vi "Generate External Actuator Channels.vi"() -> (1 "Output Channels":refnum<k21>[](array[refnum]), 3 "Input Channels":refnum<k21>[](array[refnum]))   [LabVIEW 2009]
uses:
  Data Access Objects/Metadata/Persistant DAO Actions.ctl
  Data Access Objects/External Actuators/External Actuator Id.ctl
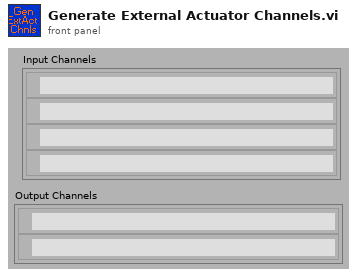
[diagram p1: front panel]
types:
  T1 = typedef "External Actuator Id.ctl" = enum16{"Left", "Right"}
  T2 = typedef "Persistant DAO Actions.ctl" = enum16{"Init", "Get", "Set", "Load", "Save"}
  T3 = typedef "External Actuator Channels.ctl" = cluster{"Load Cell":refnum<k21>, "LVDT":refnum<k21>, "Command":refnum<k21>, "Command\nReturn":refnum<k21>}
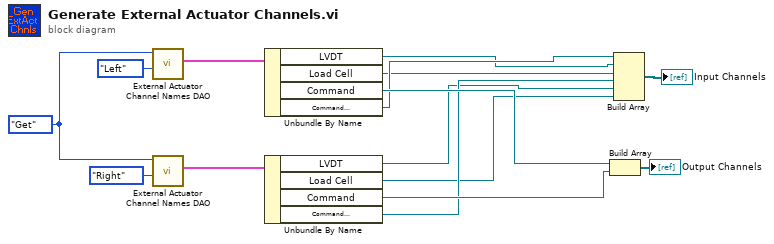
[diagram p0: block diagram]
diagram:
  w11 = Persistant_DAO_Actions."Get" ("Persistent DAO Actions")
  n1 = call "External Actuator Channel Names DAO.vi"("External Actuator Id"=External_Actuator_Id."Left", "Persistent DAO Actions"=w11) -> ("DAQ Channel Out"=w14:T3)  [unwired: 7 in, 2 out]
  n2 = call "External Actuator Channel Names DAO.vi"("External Actuator Id"=External_Actuator_Id."Right", "Persistent DAO Actions"=w11) -> ("DAQ Channel Out"=w12:T3)  [unwired: 7 in, 2 out]
  n3 = Unbundle By Name(w14) -> ("LVDT"=w5:refnum<k21>, "Load Cell"=w4:refnum<k21>, "Command"=w10:refnum<k21>, "Command\nReturn"=w6:refnum<k21>)
  n4 = Unbundle By Name(w12) -> ("LVDT"=w2:refnum<k21>, "Load Cell"=w1:refnum<k21>, "Command"=w9:refnum<k21>, "Command\nReturn"=w3:refnum<k21>)
  n5 = Build Array(w10, w9) -> (→"Output Channels":refnum<k21>[])
  n6 = Build Array(w6, w5, w4, w3, w2, w1) -> (→"Input Channels":refnum<k21>[])
